vi "add_int64.vi"   [LabVIEW 2010]
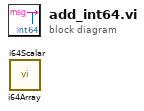
[diagram p0: block diagram]
diagram:
  n1 = call <userlib>:"i64Array.vi"() -> ()  [unwired: 5 in, 1 out]
  n2 = call <userlib>:"i64Scalar.vi"() -> ()  [unwired: 5 in, 1 out]
